vi "Clean Layout.vi"(8 "error in (no error)":errorcluster, 11 "TabCtls":refnum<vi>[](array[refnum])) -> (0 "error out":errorcluster)   [LabVIEW 2020, in "MDI ViewManager.lvlib"]
uses:
  MDI ViewManager.lvlib
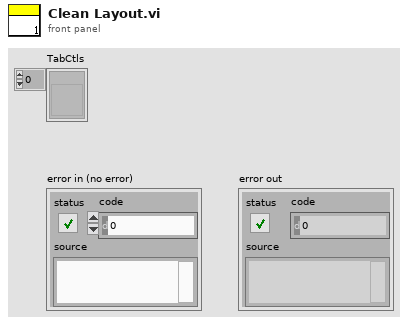
[diagram p1: front panel]
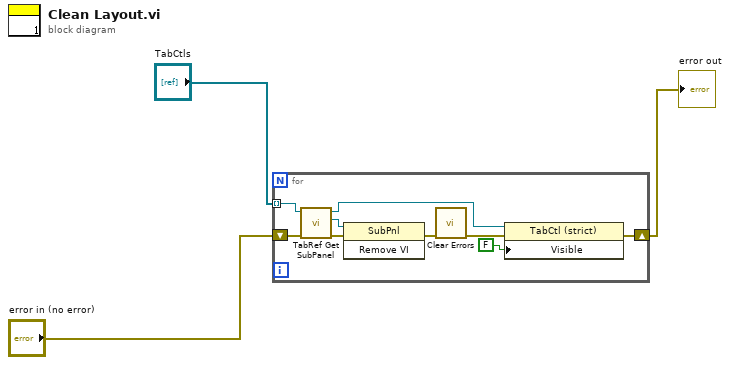
[diagram p0: block diagram]
diagram:
  n1 = for {
    tunnel: "TabCtls" -> [w8] mode=indexing
    shift-right: [w5] -> w3
    shift-left: "error in (no error)" -> [w6]
    n2 = call "TabRef Get SubPanel.vi"("error in (no error)"=w6, "TabControl in"=w8) -> ("error out"=w7:errorcluster, "Sub Panel"=w9:refnum<vi>, "TabControl out"=w4:refnum<vi>)  [unwired: 7 in]
    n3 = invoke class="SubPnl" method="Remove VI"(reference=w9, error in=w7) -> (error out=w11:errorcluster)  [unwired: 1 in, 2 out]
    n4 = call <vilib>:"Clear Errors.vi"("error in (no error)"=w11) -> ("error out"=w10:errorcluster)  [unwired: 5 in, 1 out]
    n5 = property class="TabCtl (strict)"(reference=w4, error in=w10, "Visible"=FALSE) -> (error out=w5:errorcluster)  [unwired: 1 out]
  }
  "error out" <- w3
